vi "Create Parameters Filename.vi"(0 "Simulyzer File Path":path caption="selected path", 11 "error in (no error)":errorcluster) -> (4 "Parm File Path":path caption="selected path", 15 "error out":errorcluster)   [LabVIEW 2013, in "AIT 664 Custom Device.lvlib"]
doc: "Given a xml configuration file create the corisponding parameters configuraiton file"
uses:
  AIT 664 Custom Device.lvlib
panel:
  out "lowercase file extension":string
  out "filename without extension":string
  out "stripped path":path
  out "name":string
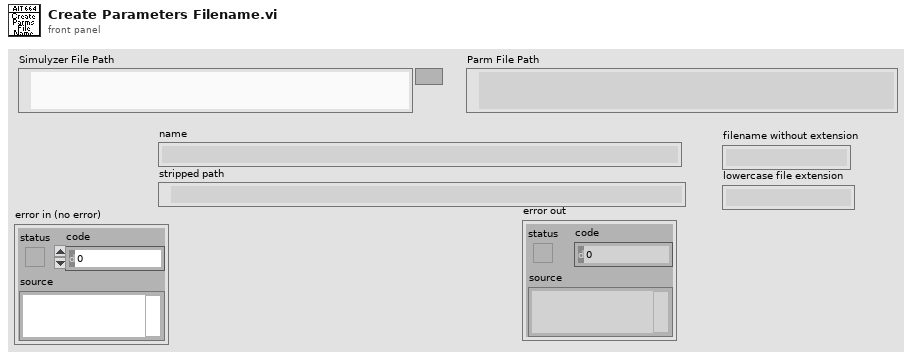
[diagram p1: front panel]
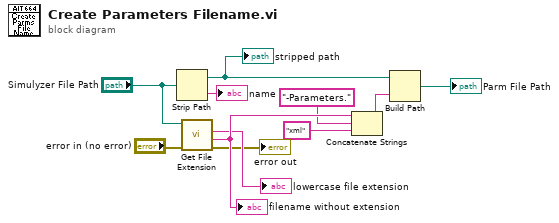
[diagram p0: block diagram]
diagram:
  n1 = Strip Path(path="Simulyzer File Path") -> (stripped path=w9:path, name=→"name":string)
  "stripped path" <- w9
  n2 = call <vilib>:"Get File Extension.vi"("error in (no error)"="error in (no error)", "file"="Simulyzer File Path") -> ("error out"=→"error out":errorcluster, "filename without extension"=w7:string, "lowercase file extension"=→"lowercase file extension":string)  [unwired: 6 in, 1 out]
  "filename without extension" <- w7
  n3 = Concatenate Strings(w7, "-Parameters." ("string"), "xml" ("string")) -> (w5:string)
  n4 = Build Path(base path=w9, name or relative path=w5) -> (appended path=→"Parm File Path":path)
